vi "Viewer.vi"() -> ()   [LabVIEW 2018]
panel:
  out "XY Graph":cluster{i32[], i32[]}[](graph)
  in  "Select Result":path
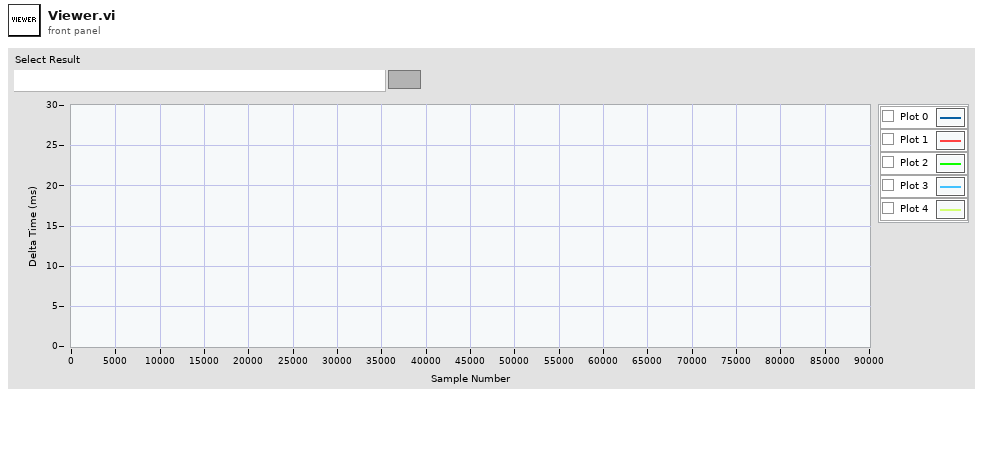
[diagram p1: front panel]
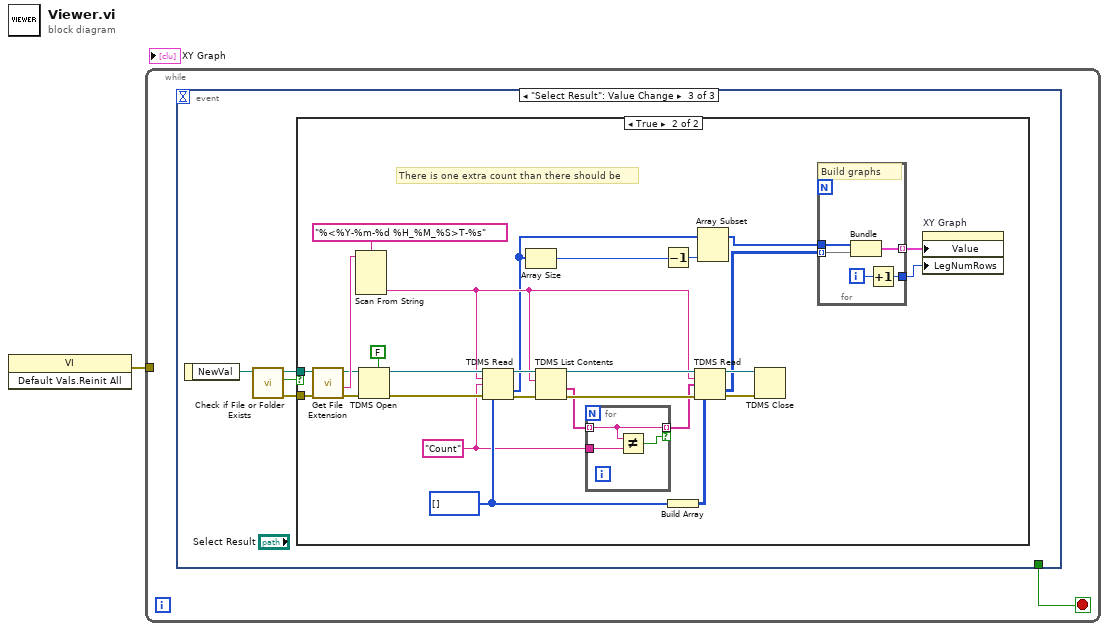
[diagram p0: block diagram]
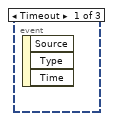
[diagram p2: hidden frame]
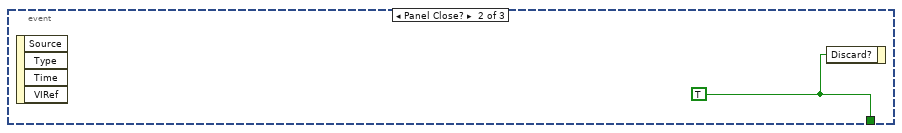
[diagram p3: hidden frame]
diagram:
  n1 = invoke class="VI" method="Default Vals.Reinit All"() -> (error out=w1:errorcluster)  [unwired: 3 in, 2 out]
  n2 = while {
    tunnel: w1 -> [_]
    stop <- w2 stop-if-true
    n3 = event shown="[2] \"Select Result\": Value Change" {
      selector: _ -> [_ _ _]
      dyn-events: _ -> [_ _ _]
      timeout: _ -> [_ _ _]
      tunnel: [_ w3 _] -> w2
      event Timeout {
        n4 = event-data() -> ()  [unwired: 1 in, 3 out]
      }
      event Panel Close? {
        w3 = TRUE
        n5 = event-data() -> ()  [unwired: 1 in, 4 out]
        n6 = event-data("Discard?"=w3) -> ()  [unwired: 1 in, 1 out]
      }
      event "Select Result": Value Change {
        n7 = event-data() -> ("NewVal"=w7:path)  [unwired: 1 in]
        n8 = call <vilib>:"Check if File or Folder Exists.vi"("path"=w7) -> ("error out"=w4:errorcluster, "file or folder exists?"=w5:bool, "dup path"=w6:path)  [unwired: 8 in]
        n9 = case shown="True" w5 {
          tunnel: w6 -> [_ w33]
          tunnel: w4 -> [_ w30]
          frame False {
          }
          frame True {
            w20 = i32[] []
            w9 = "Count"
            # "There is one extra count than there should be"
            n10 = call <vilib>:"Get File Extension.vi"("error in (no error)"=w30, "file"=w33) -> ("error out"=w31:errorcluster, "filename without extension"=w32:string, "dup file"=w29:path)  [unwired: 5 in, 2 out]
            n11 = Scan From String(format string="%<%Y-%m-%d %H_%M_%S>T-%s", input string=w32) -> (output 2=w21:string)  [unwired: 5 in, 3 out]
            n12 = TDMS Open(5:FALSE ("create index file? (T)"), 8:w31, 11:w29) -> (0:w26:errorcluster, 3:w27:refnum<k34>)  [unwired: 4 in]
            n13 = TDMS Read(0:w27, 5:w21, 7:w9, 11:w26, 12:w20) -> (4:w25:refnum<k34>, 10:w12:i32[], 15:w24:errorcluster)  [unwired: 3 in, 3 out]
            n14 = Array Size(array=w12) -> (size(s)=w14:i32)
            n15 = TDMS List Contents(4:w24, 6:w21, 7:w25) -> (0:w23:errorcluster, 1:w11:string[], 3:w22:refnum<k34>)  [unwired: 1 out]
            n16 = for {
              tunnel: w11 -> [w42] mode=indexing
              tunnel: [w42] -> w10 mode=indexing if=w41
              tunnel: w9 -> [w40]
              n17 = Not Equal?(x=w42, y=w40) -> (x != y?=w41:bool)
            }
            n18 = Decrement(x=w14) -> (x-1=w13:i32)
            n19 = Build Array(w20) -> (w19:i32[][])
            n20 = TDMS Read(0:w22, 5:w21, 7:w10, 11:w23, 12:w19) -> (4:w18:refnum<k34>, 10:w16:i32[][], 15:w17:errorcluster)  [unwired: 3 in, 3 out]
            n21 = Array Subset(array=w12, length=w13) -> ()  [unwired: 1 in, 1 out]
            n22 = TDMS Close(8:w17, 11:w18) -> ()  [unwired: 2 out]
            n23 = for {
              tunnel: w16 -> [w35] mode=indexing
              tunnel: w12 -> [w39]
              tunnel: [w38] -> w15 mode=indexing
              tunnel: [w36] -> w8
              i -> [w37]
              # "Build graphs"
              n24 = Bundle(w39, w35) -> (w38:cluster{i32[], i32[]})  [unwired: 1 in]
              n25 = Increment(x=w37) -> (x+1=w36:i32)
            }
            n26 = property on="XY Graph" class="XYGraph (strict)"("Value"=w15, "LegNumRows"=w8) -> ()  [unwired: 2 in, 2 out]
          }
        }
      }
    }
  }
